vi "2100_SP3T_SMU_Source and Sink_Meas and Calc Resistance.vi"(7 "Current  Level":dbl=-0.01 format="%#_6p", 8 "error in (no error)":errorcluster, 10 "Pins":string[](array[string]), 11 "Semiconductor Module Context":T1) -> (0 "error Out":errorcluster, 1 "Avg_Parallel_Calc":dbl[](array[numeric]), 2 "Avg_Individual_Throws":dbl[](array[numeric]), 3 "Semiconductor Module Context Out":T1)   [LabVIEW 2013]
uses:
  <vilib>/NI_TestStand_SemiconductorModule/NI_TestStand_Semiconductor_Module.lvlibp/PinMap/General/SemiconductorModuleContext.ctl
  <vilib>/NI_TestStand_SemiconductorModule/NI_TestStand_Semiconductor_Module.lvlibp/PinMap/DC Power/PinsToNIDCPowerSessions.vi
  <vilib>/NI_TestStand_SemiconductorModule/NI_TestStand_Semiconductor_Module.lvlibp
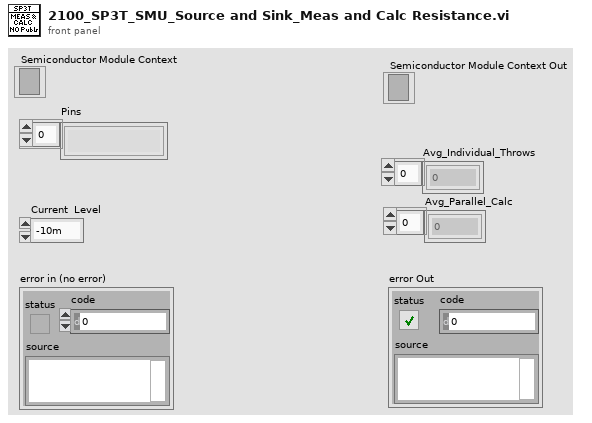
[diagram p1: front panel]
types:
  T1 = typedef "NI_TestStand_Semiconductor_Module.lvlibp/SemiconductorModuleContext.ctl" = refnum<k7>
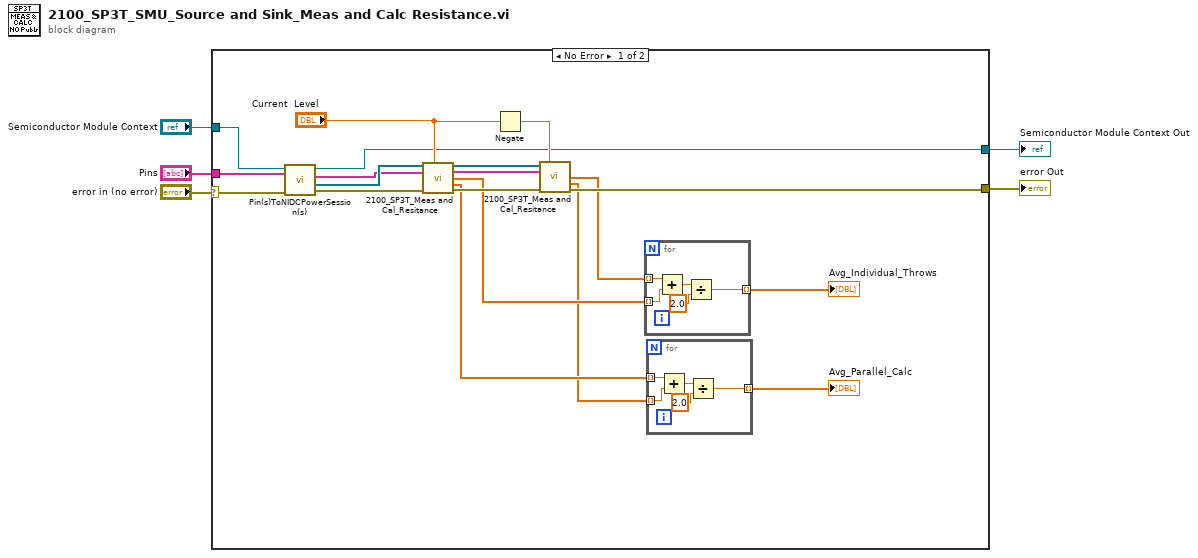
[diagram p0: block diagram]
diagram:
  n1 = case shown="No Error" "error in (no error)" {
    selector: "error in (no error)" -> [w24 w36]
    tunnel: "Semiconductor Module Context" -> [w22 w35]
    tunnel: "Pins" -> [w23 _]
    tunnel: [w13 w36] -> w2
    tunnel: [w12 w35] -> w1
    frame No Error {
      n2 = call-poly <vilib>:"Pin(s)ToNIDCPowerSession(s).vi"("error in (no error)"=w24, "Pins"=w23, "Semiconductor Module Context"=w22) -> ("error out"=w21:errorcluster, "Instrument Sessions"=w20:refnum<k15>[], "Channel Lists"=w19:string[], "Semiconductor Module Context Out"=w12:T1)  [unwired: 4 in, 1 out]
      n3 = call "2100_SP3T_Meas and Cal_Resitance.vi"("Instrument Sessions"=w20, "Current  Level"="Current  Level", "Channel Lists"=w19, "error in (no error)"=w21) -> ("Instrument Sessions out"=w15:refnum<k15>[], "Channel Lists Out"=w14:string[], "Individual_Resitances"=w10:dbl[], "Parallel_Resitance"=w9:dbl[], "error out"=w18:errorcluster)  [unwired: 7 in]
      n4 = Negate(x="Current  Level") -> (-x=w17:dbl)
      n5 = call "2100_SP3T_Meas and Cal_Resitance.vi"("Instrument Sessions"=w15, "Current  Level"=w17, "Channel Lists"=w14, "error in (no error)"=w18) -> ("Individual_Resitances"=w11:dbl[], "Parallel_Resitance"=w8:dbl[], "error out"=w13:errorcluster)  [unwired: 7 in, 2 out]
      n6 = for {
        tunnel: w11 -> [w34] mode=indexing
        tunnel: w10 -> [w33] mode=indexing
        tunnel: [w30] -> w7 mode=indexing
        n7 = Add(x=w34, y=w33) -> (x+y=w32:dbl)
        n8 = Divide(x=w32, y=2.0) -> (x/y=w30:dbl)
      }
      "Avg_Individual_Throws" <- w7
      n9 = for {
        tunnel: w9 -> [w29] mode=indexing
        tunnel: w8 -> [w28] mode=indexing
        tunnel: [w25] -> w6 mode=indexing
        n10 = Add(x=w29, y=w28) -> (x+y=w27:dbl)
        n11 = Divide(x=w27, y=2.0) -> (x/y=w25:dbl)
      }
      "Avg_Parallel_Calc" <- w6
    }
    frame Error {
    }
  }
  "error Out" <- w2
  "Semiconductor Module Context Out" <- w1
